vi "Create AI Pressure Channel.vi"(8 "error in (no error)":errorcluster, 9 "Physical channel":string, 10 "Name":string, 11 "Task in":refnum<k21>) -> (0 "error out":errorcluster, 2 "Pressure Channel Settings":string, 3 "Task out":refnum<k21>)   [LabVIEW 2021, in "Load Frame.lvlib"]
uses:
  Load Frame.lvlib
  <vilib>/DAQmx/create/channels.llb/DAQmx Create Channel (AI-Pressure-Bridge-Two-Point-Linear).vi
  <resource>/objmgr/daqmx.rc
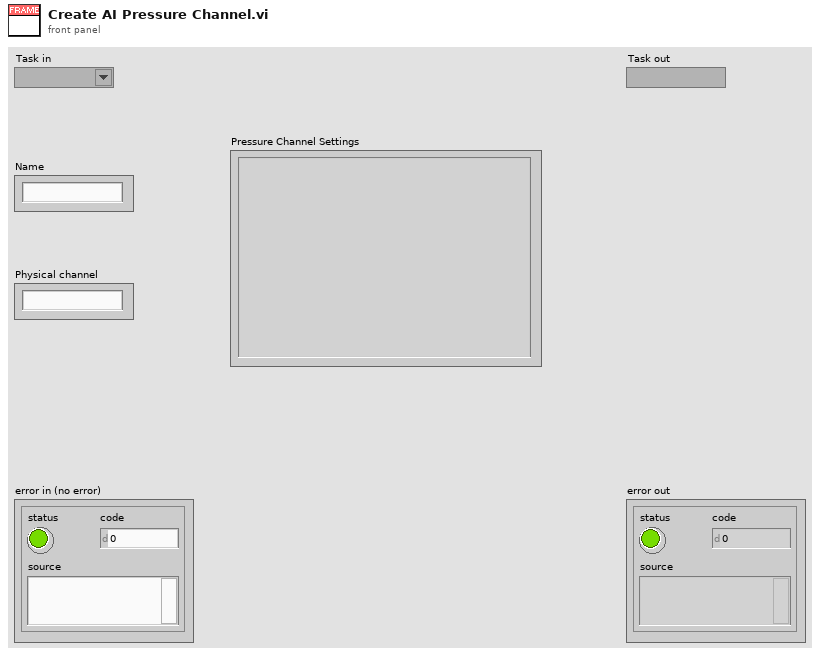
[diagram p1: front panel]
types:
  T1 = cluster{"Name":string, "Physical channel":string, "AI.Max":dbl, "AI.Min":dbl, "AI.MeasType":i32, "AI.Bridge.Cfg":i32, "AI.Bridge.NomResistance":dbl, "AI.ADCTimingMode":i32, "AI.Excit.Src":i32, "AI.Excit.Val":dbl}
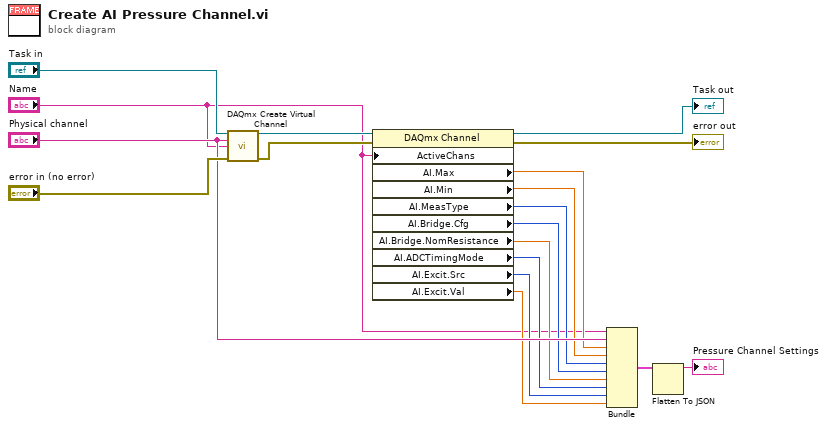
[diagram p0: block diagram]
diagram:
  n1 = call-poly <vilib>:"DAQmx Create Virtual Channel.vi"("task in"="Task in", "physical channels"="Physical channel", "name to assign"="Name", "error in"="error in (no error)") -> ("task out"=w17:refnum<k21>, "error out"=w14:errorcluster)  [unwired: 10 in]
  n2 = property class="DAQmx Channel"(reference=w17, error in=w14, "ActiveChans"="Name") -> (reference out=→"Task out":refnum<k21>, error out=→"error out":errorcluster, "AI.Max"=w10:dbl, "AI.Min"=w9:dbl, "AI.MeasType"=w8:i32, "AI.Bridge.Cfg"=w7:i32, "AI.Bridge.NomResistance"=w6:dbl, "AI.ADCTimingMode"=w5:i32, "AI.Excit.Src"=w4:i32, "AI.Excit.Val"=w3:dbl)
  n3 = Bundle("Name"="Name", "Physical channel"="Physical channel", "AI.Max"=w10, "AI.Min"=w9, "AI.MeasType"=w8, "AI.Bridge.Cfg"=w7, "AI.Bridge.NomResistance"=w6, "AI.ADCTimingMode"=w5, "AI.Excit.Src"=w4, "AI.Excit.Val"=w3) -> (w12:T1)  [unwired: 1 in]
  n4 = Flatten To JSON(anything=w12) -> (JSON string=→"Pressure Channel Settings":string)  [unwired: 2 in, 1 out]
